vi "TEST_IR_OPO_Capture_V2.vi"(3 "AD status":bool, 5 "XPS_Address":string="192.168.254.254", 7 "laser array index":i32, 8 "OPO on?":bool, 9 "Process time":dbl format="%#_13g", 11 "Axis Speed":dbl=1.0 format="%#_13g", 12 "stop":bool, 13 "Axis Initial Parameters":T1={"Velocity (units/seconds)"=1.0, "Acceleration (units/seconds²)"=20.0, "Minimum Jerk Time (seconds)"=0.005, "Maximum Jerk Time (seconds)"=0.009} {"Maximum Jerk Time (seconds)" format="%.6e"; "Minimum Jerk Time (seconds)" format="%.6e"; "Acceleration (units/seconds²)" format="%.6e"; "Velocity (units/seconds)" format="%.6e"}, 14 "ROI Area \n(mm2)":dbl=4.035870075999999, 15 "Acceleration (units/seconds²)":dbl=20.0) -> (2 "Elapsed time":dbl)   [LabVIEW 2016]
uses:
  case selector.ctl
panel:
  in  "Commands array":string[][](array[string])=[["Group31.000000", "Group20.100000"], ["Group3-1.000000", "Group20.100000"], ["Group31.000000", "Group20.100000"], ["Group3-1.000000", "Group20.100000"], ["Group31.000000", "Group20.100000"], ["Group3-1.000000", "Group20.100000"], ["Group31.000000", "Group20.100000"], ["Group3-1.000000", "Group20.100000"], ["Group31.000000", "Group20.100000"], ["Group3-1.000000", "Group20.100000"], ["Group31.000000", "Group20.100000"], ["Group3-1.000000", "Group20.100000"]]
  in  "Laser on/off array":bool[][](array[boolean])=[[TRUE, FALSE], [TRUE, FALSE], [TRUE, FALSE], [TRUE, FALSE], [TRUE, FALSE], [TRUE, FALSE], [TRUE, FALSE], [TRUE, FALSE], [TRUE, FALSE], [TRUE, FALSE], [TRUE, FALSE], [TRUE, FALSE]]
  out "Capture Log":string="ROI Area (mm2) = 4.035870Axis 1 = 30.733482  -  Axis 2 = 11.861419\r"
  out "Axis 1 position":dbl=30.73348220365 format="%.10f"
  out "Axis 2 position":dbl=11.86141924161 format="%.10f"
  out "Initial time":timestamp=timestamp(3577899423.208551 s since 1904-01-01)
  in  "Active Positioner":string="Group2.Pos"
  out "Current Line":i32
  out "1D Laser Array":bool[](array[boolean])=[TRUE, FALSE, TRUE, FALSE, TRUE, FALSE, TRUE, FALSE, TRUE, FALSE, TRUE, FALSE, TRUE, FALSE, TRUE, FALSE, TRUE, FALSE, TRUE, FALSE, TRUE, FALSE, TRUE, FALSE]
  out "1D command array":string[](array[string])=["Group31.068", "Group20.084", "Group3-1.068", "Group20.084", "Group31.068", "Group20.084", "Group3-1.068", "Group20.084", "Group31.068", "Group20.084", "Group3-1.068", "Group20.084", "Group31.068", "Group20.084", "Group3-1.068", "Group20.084", "Group31.068", "Group20.084", "Group3-1.068", "Group20.084", "Group31.068", "Group20.084", "Group3-1.068", "Group20.084"]
  out "Current Command":string
  out "Current laser element":bool
  out "Total lines":i32
  in  "Active Axis":string="Group2"
  out "Laser on/off":bool
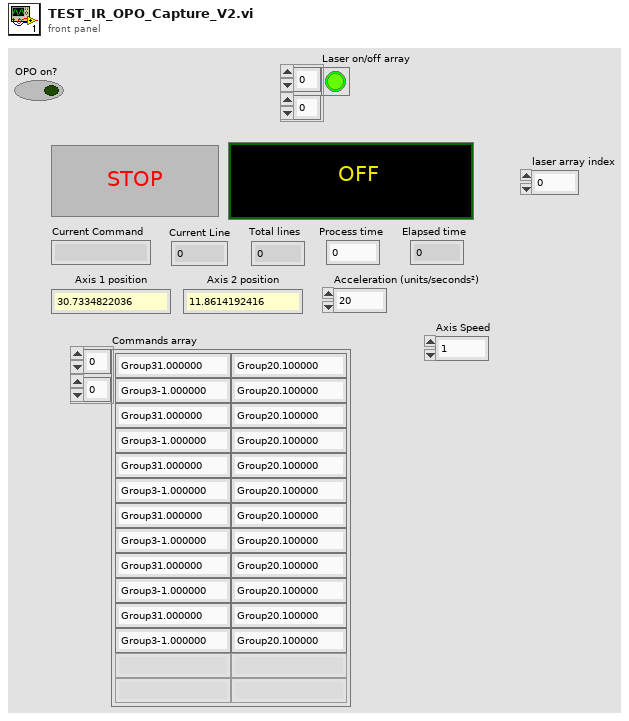
[diagram p1: front panel]
types:
  T1 = cluster{"Velocity (units/seconds)":dbl, "Acceleration (units/seconds²)":dbl, "Minimum Jerk Time (seconds)":dbl, "Maximum Jerk Time (seconds)":dbl}
  T2 = typedef "case selector.ctl" = enum16{"Initialize", "Element selection", "Laser", "Velocities", "Command", "Wait", "Exit"}
  T3 = enum16{"Initialize", "Lamp ON", "Lamp OFF", "Q-switch ON", "Q-switch OFF", "Adjust Energy", "Change Rep. Rate", "Send String"}
  T4 = enum16{"open", "replace", "create", "open or create", "replace or create", "replace or create with confirmation"}
  T5 = cluster{"connection TCP":refnum<k5>, "LogTo File":bool, "Log File refnum":refnum<file>, "no error if error log":bool}
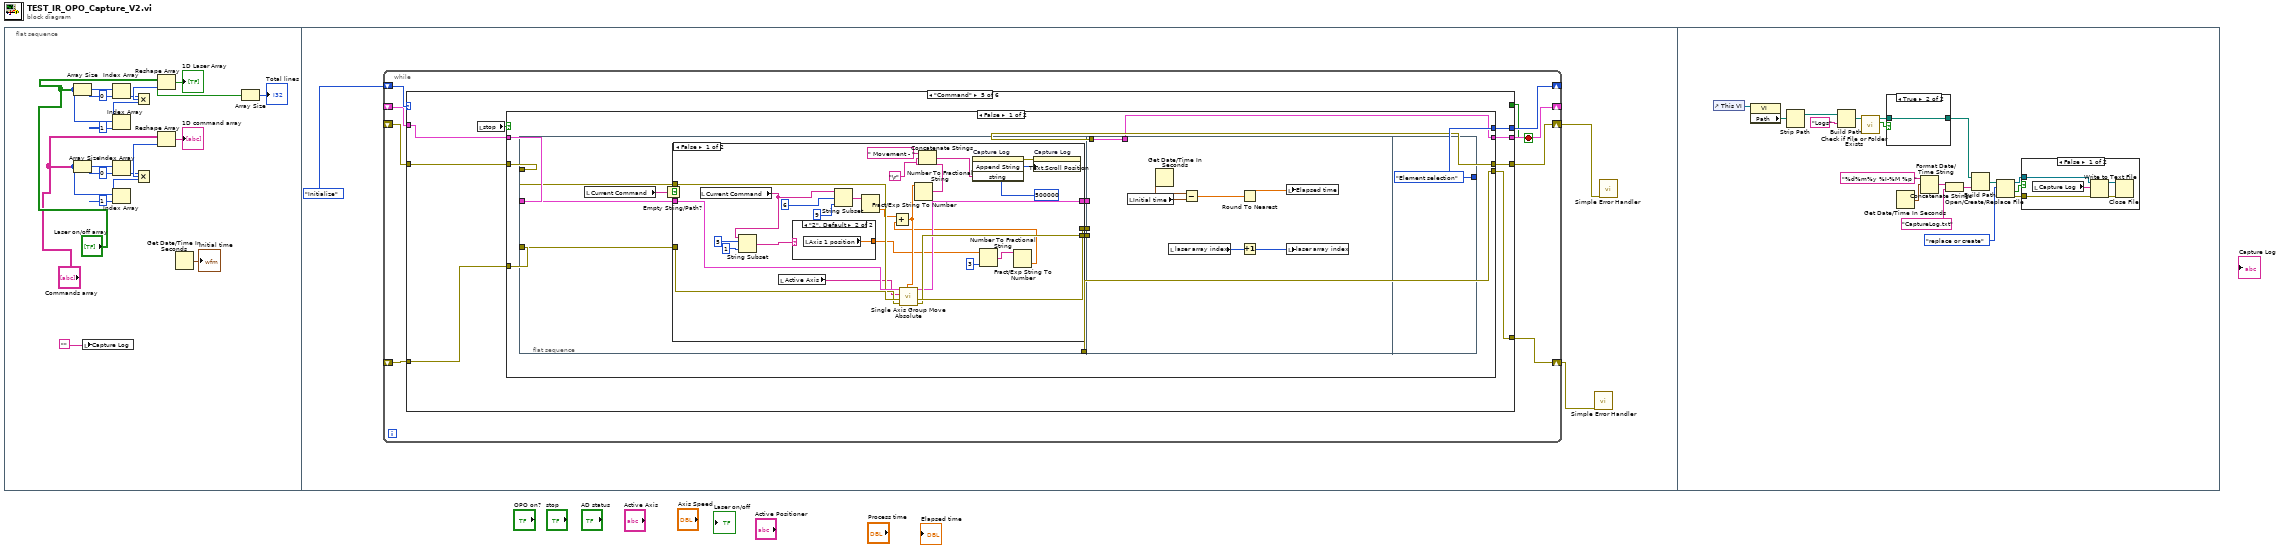
[diagram p0: block diagram]
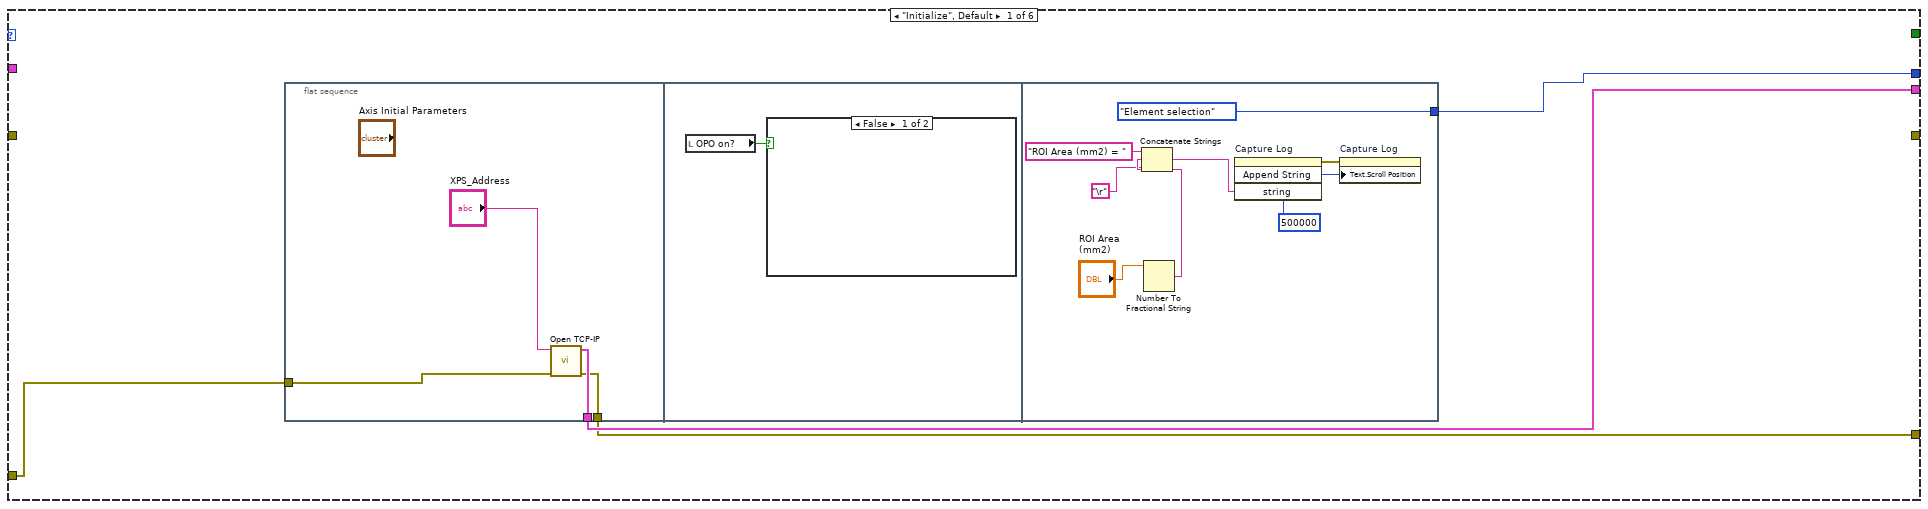
[diagram p2: hidden frame]
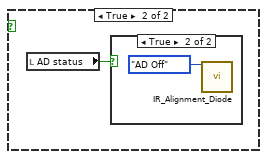
[diagram p3: hidden frame]
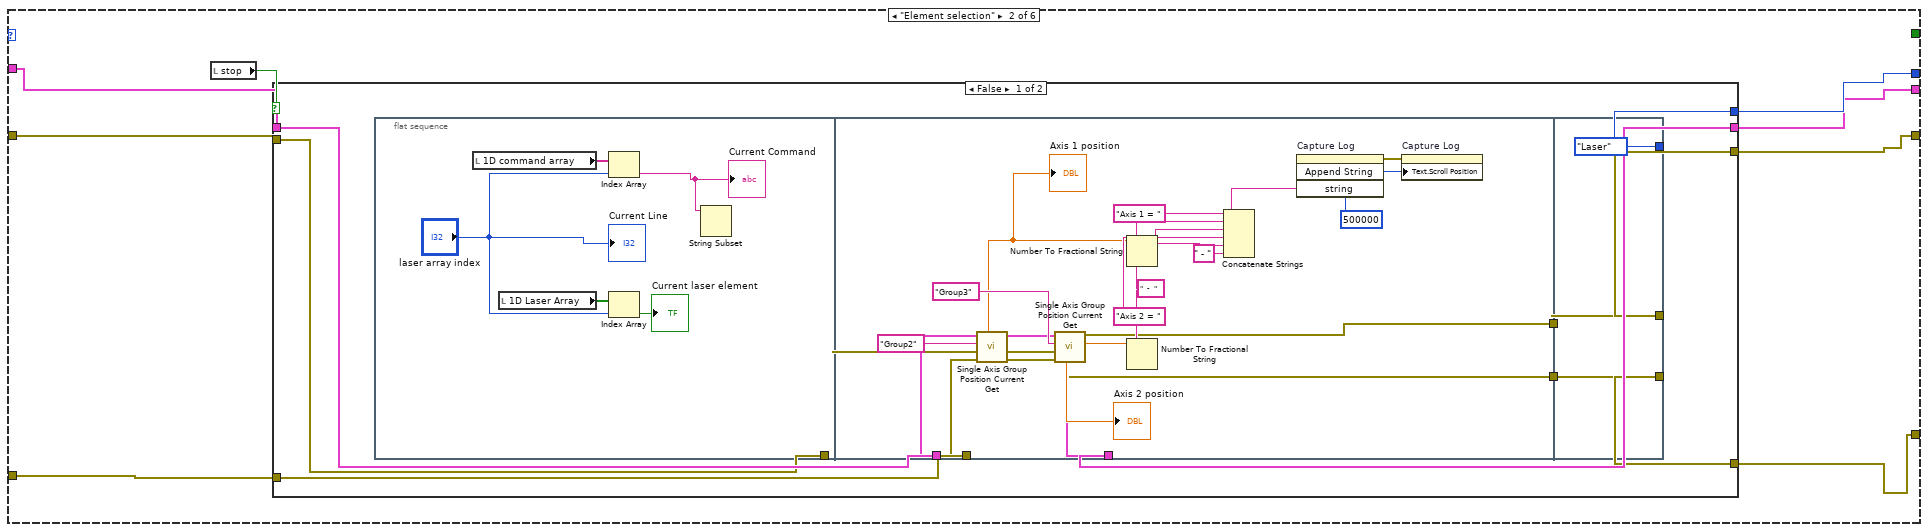
[diagram p5: hidden frame]
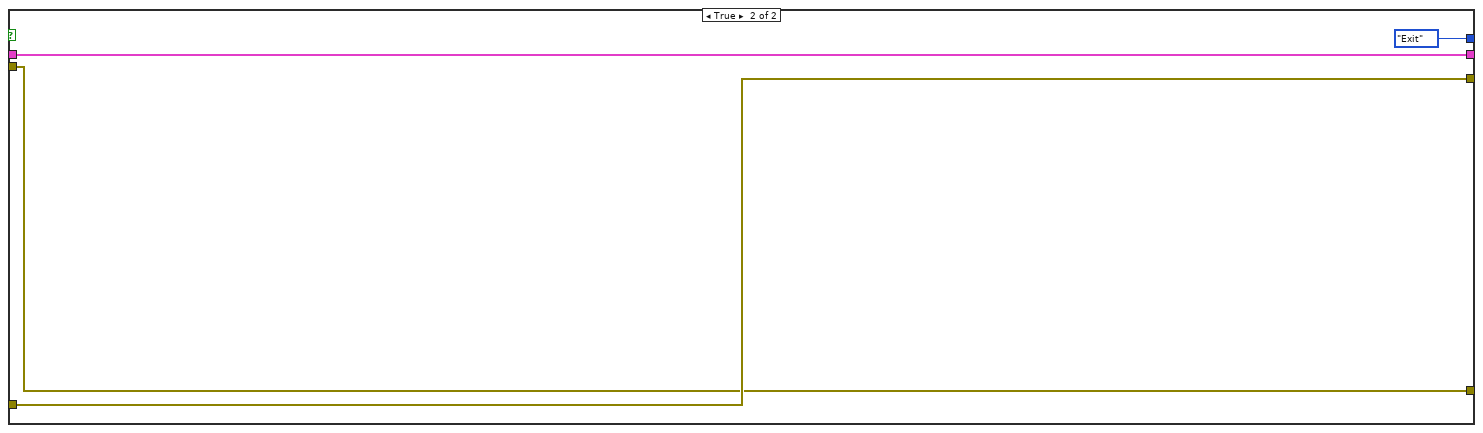
[diagram p6: hidden frame]
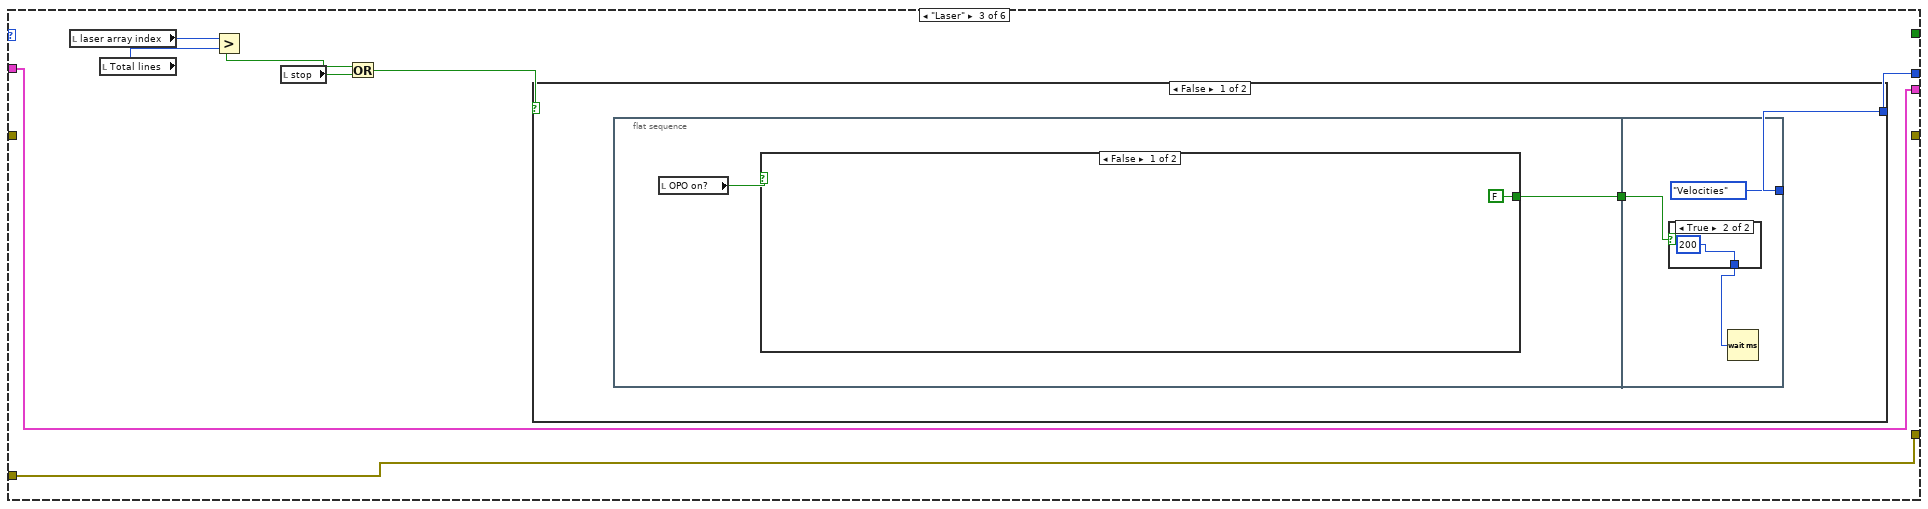
[diagram p7: hidden frame]
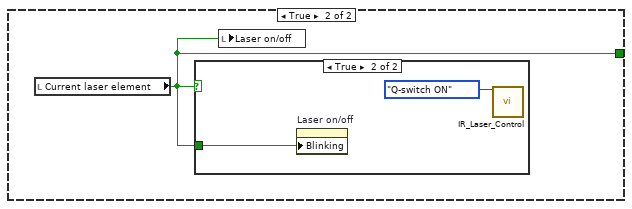
[diagram p8: hidden frame]
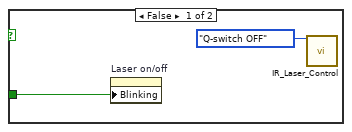
[diagram p9: hidden frame]
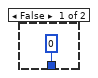
[diagram p10: hidden frame]
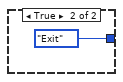
[diagram p11: hidden frame]
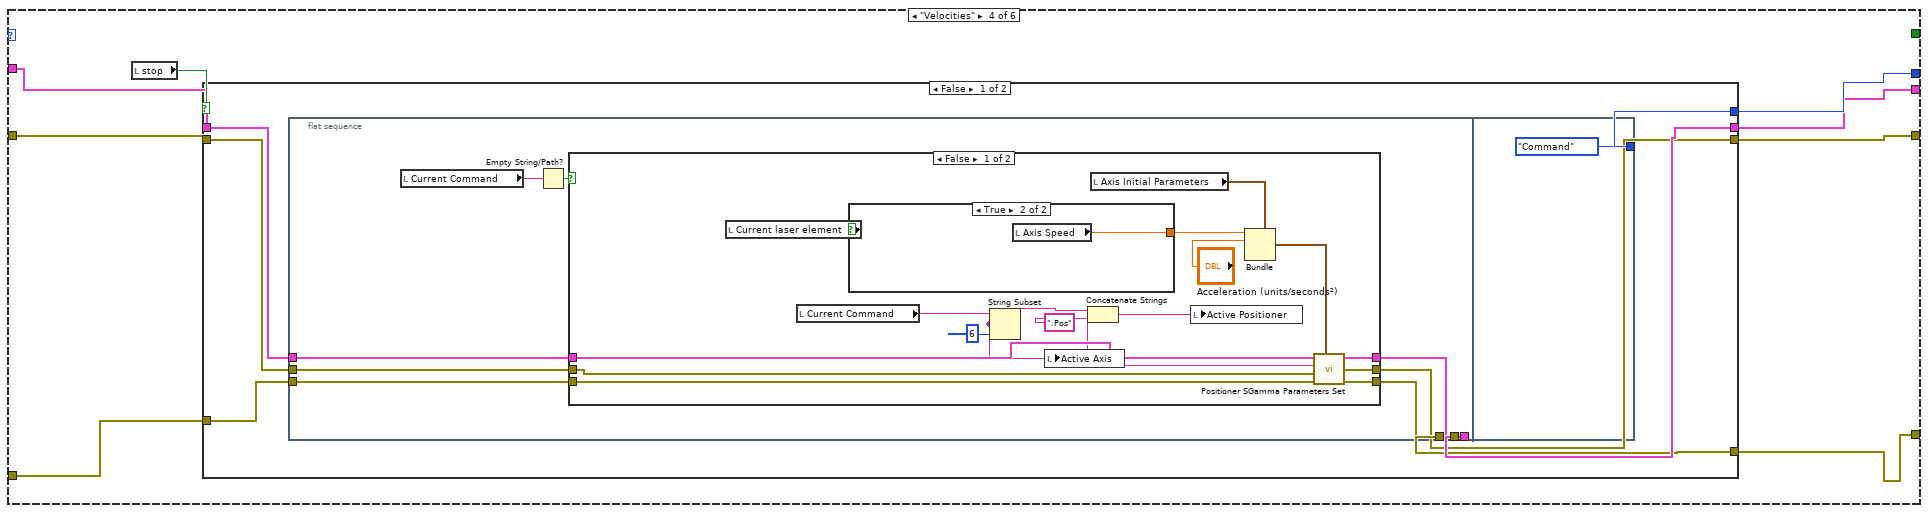
[diagram p12: hidden frame]
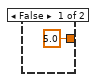
[diagram p13: hidden frame]
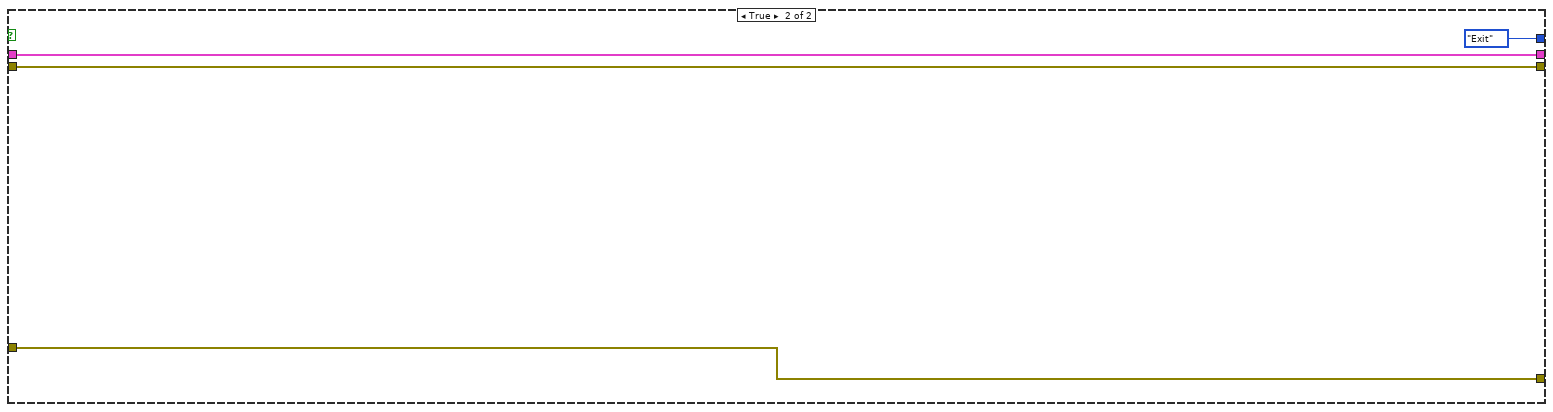
[diagram p15: hidden frame]
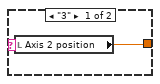
[diagram p16: hidden frame]
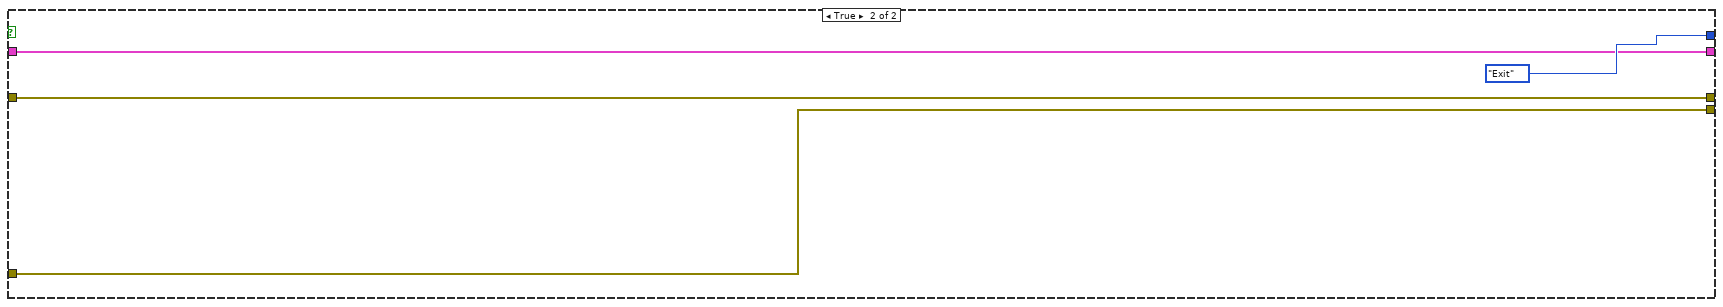
[diagram p18: hidden frame]
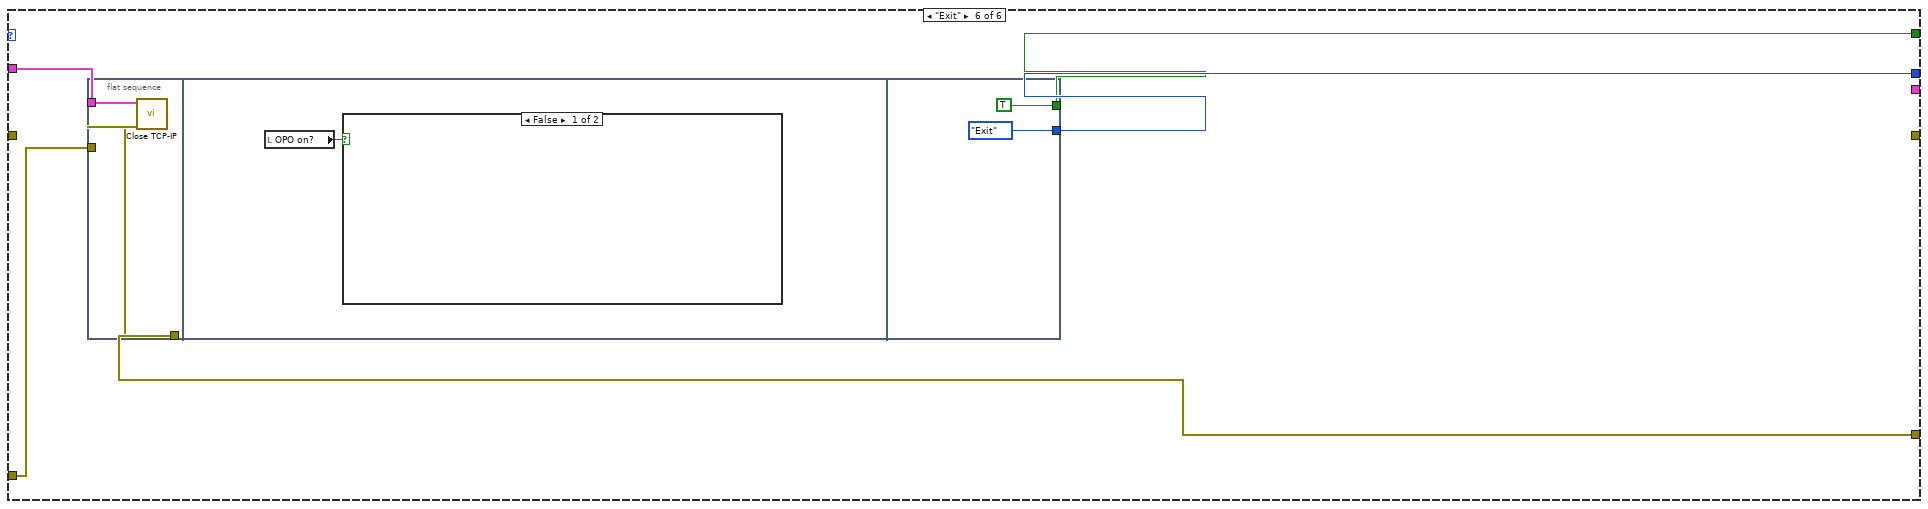
[diagram p19: hidden frame]
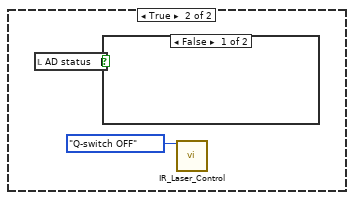
[diagram p20: hidden frame]
diagram:
  n1 = flat-sequence {
    frame #0 {
      n2 = Array Size(array="Laser on/off array") -> (size(s)=w12:i32[])
      n3 = Array Size(array="Commands array") -> (size(s)=w5:i32[])
      n4 = local write "Capture Log"("") -> ()
      n5 = Index Array(array=w12, index=0) -> (element=w15:i32)
      n6 = Index Array(array=w12, index=1) -> (element=w16:i32)
      n7 = Index Array(array=w5, index=0) -> (element=w8:i32)
      n8 = Index Array(array=w5, index=1) -> (element=w9:i32)
      n9 = Multiply(x=w15, y=w16) -> (x*y=w17:i32)
      n10 = Multiply(x=w8, y=w9) -> (x*y=w10:i32)
      n11 = Reshape Array("Laser on/off array", w17) -> (w19:bool[])
      "1D Laser Array" <- w19
      n12 = Reshape Array("Commands array", w10) -> (→"1D command array":string[])
      n13 = Get Date/Time In Seconds() -> (seconds since 1Jan1904=→"Initial time":timestamp)
      n14 = Array Size(array=w19) -> (size(s)=→"Total lines":i32)
    }
    frame #1 {
      n15 = while {
        shift-right: [w30] -> _
        shift-left: case_selector."Initialize" -> [w31]
        shift-right: [w28] -> w20
        shift-left: _ -> [w29]
        shift-right: [w27] -> _
        shift-left: _ -> [w26]
        shift-right: [w25] -> w21
        shift-left: _ -> [w24]
        stop <- w23 stop-if-true
        n16 = case shown="\"Command\"" w31 {
          tunnel: [w35 w58 w109 w133 w182 w247] -> w30
          tunnel: w29 -> [w34 w55 w108 w131 w180 w248]
          tunnel: [w32 w52 w108 w130 w179 w246] -> w28
          tunnel: [w33 w51 w102 w128 w177 _] -> w27
          tunnel: w26 -> [_ w56 w102 w129 w178 w245]
          tunnel: [_ w53 _ w127 w175 _] -> w25
          tunnel: w24 -> [_ w54 _ w126 w176 _]
          tunnel: [_ _ _ _ _ w244] -> w23
          frame "Initialize", Default {
            n17 = flat-sequence {
              tunnel: w34 -> [w38]
              tunnel: [w37] -> w33
              tunnel: [w36] -> w32
              tunnel: [case_selector."Element selection"] -> w35
              frame #0 {
                n18 = call <userlib>:"Open TCP-IP.vi"("error in (no error)"=w38, "IP address"="XPS_Address") -> ("error out"=w36:errorcluster, "Connection ID"=w37:T5)  [unwired: 7 in, 1 out]
              }
              frame #1 {
                n19 = local read "OPO on?"() -> (w40:bool)
                n20 = case shown="False" w40 {
                  frame False {
                  }
                  frame True {
                    n21 = local read "AD status"() -> (w41:bool)
                    n22 = case shown="True" w41 {
                      frame False {
                      }
                      frame True {
                        n23 = call "IR_Alignment_Diode.vi"("AD Action"=enum16{"AD Off", "AD On"}."AD Off") -> ()  [unwired: 14 in, 1 out]
                      }
                    }
                  }
                }
              }
              frame #2 {
                n24 = Number To Fractional String(number="ROI Area \n(mm2)") -> (F-format string=w46:string)  [unwired: 3 in]
                n25 = Concatenate Strings("ROI Area (mm2) = " ("string"), w46, "\r") -> (w44:string)
                n26 = invoke on="Capture Log" class="Str" method="Append String"("string"=w44) -> (error out=w48:errorcluster)  [unwired: 3 in, 3 out]
                n27 = property on="Capture Log" class="Str"(error in=w48, "Text.Scroll Position"=u32 500000) -> ()  [unwired: 1 in, 2 out]
              }
            }
          }
          frame "Element selection" {
            n28 = local read "stop"() -> (w57:bool)
            n29 = case shown="False" w57 {
              tunnel: [w64 case_selector."Exit"] -> w58
              tunnel: w56 -> [w67 w100]
              tunnel: w55 -> [w66 w99]
              tunnel: w54 -> [w65 w98]
              tunnel: [w59 w99] -> w53
              tunnel: [w61 w98] -> w52
              tunnel: [w63 w100] -> w51
              frame False {
                n30 = flat-sequence {
                  tunnel: w67 -> [w86]
                  tunnel: w66 -> [w84]
                  tunnel: w65 -> [w83]
                  tunnel: [w76] -> w63
                  tunnel: [w75] -> w62
                  tunnel: [w74] -> w60
                  tunnel: [case_selector."Laser"] -> w64
                  tunnel: w62 -> [w96]
                  tunnel: [w96] -> w61
                  tunnel: w60 -> [w95]
                  tunnel: [w95] -> w59
                  frame #0 {
                    n31 = local read "1D command array"() -> (w71:string[])
                    n32 = local read "1D Laser Array"() -> (w70:bool[])
                    n33 = Index Array(array=w71, index="laser array index") -> (element=w68:string)
                    "Current Command" <- w68
                    n34 = Index Array(array=w70, index="laser array index") -> (element=→"Current laser element":bool)
                    n35 = String Subset(string=w68) -> ()  [unwired: 2 in, 1 out]
                    "Current Line" <- "laser array index"
                  }
                  frame #1 {
                    n36 = call <userlib>:"Single Axis Group Position Current Get.vi"("error in (no error)"=w84, "XPS error in (no error)"=w83, "SingleAxis Group  Name (250 c max)"="Group2" ("Axis 1"), "connection ID in"=w86) -> ("error out"=w77:errorcluster, "XPS error out"=w78:errorcluster, "Current Position (units)"=w82:dbl, "connection ID out"=w79:T5)  [unwired: 4 in]
                    "Axis 1 position" <- w82
                    n37 = call <userlib>:"Single Axis Group Position Current Get.vi"("error in (no error)"=w77, "XPS error in (no error)"=w78, "SingleAxis Group  Name (250 c max)"="Group3" ("Axis 2"), "connection ID in"=w79) -> ("error out"=w75:errorcluster, "XPS error out"=w74:errorcluster, "Current Position (units)"=w81:dbl, "connection ID out"=w76:T5)  [unwired: 4 in]
                    "Axis 2 position" <- w81
                    n38 = Number To Fractional String(number=w82) -> (F-format string=w93:string)  [unwired: 3 in]
                    n39 = Number To Fractional String(number=w81) -> (F-format string=w91:string)  [unwired: 3 in]
                    n40 = Concatenate Strings("Axis 1 = " ("string"), w93, "  -  " ("string"), "Axis 2 = " ("string"), w91, " - " ("string")) -> (w89:string)
                    n41 = invoke on="Capture Log" class="Str" method="Append String"("string"=w89) -> (error out=w88:errorcluster)  [unwired: 3 in, 3 out]
                    n42 = property on="Capture Log" class="Str"(error in=w88, "Text.Scroll Position"=u32 500000) -> ()  [unwired: 1 in, 2 out]
                  }
                  frame #2 {
                  }
                }
              }
              frame True {
              }
            }
          }
          frame "Laser" {
            n43 = local read "laser array index"() -> (w106:i32)
            n44 = local read "Total lines"() -> (w107:i32)
            n45 = Greater?(x=w106, y=w107) -> (0:w104:bool)
            n46 = local read "stop"() -> (w105:bool)
            n47 = Or(x=w104, y=w105) -> (x .or. y?=w103:bool)
            n48 = case shown="False" w103 {
              tunnel: [w111 case_selector."Exit"] -> w109
              frame False {
                n49 = flat-sequence {
                  tunnel: [w112] -> w110
                  tunnel: [case_selector."Velocities"] -> w111
                  tunnel: w110 -> [w120]
                  frame #0 {
                    n50 = local read "OPO on?"() -> (w113:bool)
                    n51 = case shown="False" w113 {
                      tunnel: [FALSE ("Current laser element") w115] -> w112
                      frame False {
                      }
                      frame True {
                        n52 = local read "Current laser element"() -> (w115:bool)
                        n53 = case shown="True" w115 {
                          tunnel: w115 -> [w116 w118]
                          frame False {
                            n54 = property on="Laser on/off" class="Bool (strict)"("Blinking"=w116) -> ()  [unwired: 2 in, 2 out]
                            n55 = call "IR_Laser_Control.vi"("Action"=T3."Q-switch OFF") -> ()  [unwired: 14 in, 1 out]
                          }
                          frame True {
                            n56 = property on="Laser on/off" class="Bool (strict)"("Blinking"=w118) -> ()  [unwired: 2 in, 2 out]
                            n57 = call "IR_Laser_Control.vi"("Action"=T3."Q-switch ON") -> ()  [unwired: 14 in, 1 out]
                          }
                        }
                        n58 = local write "Laser on/off"(w115) -> ()
                      }
                    }
                  }
                  frame #1 {
                    n59 = case shown="True" w120 {
                      tunnel: [u32 0 ("milliseconds to wait") u32 200 ("milliseconds to wait")] -> w121
                      frame False {
                      }
                      frame True {
                      }
                    }
                    n60 = Wait (ms)(milliseconds to wait=w121) -> ()  [unwired: 1 out]
                  }
                }
              }
              frame True {
              }
            }
          }
          frame "Velocities" {
            n61 = local read "stop"() -> (w132:bool)
            n62 = case shown="False" w132 {
              tunnel: [w140 case_selector."Exit"] -> w133
              tunnel: w131 -> [w139 w173]
              tunnel: [w136 w173] -> w130
              tunnel: w129 -> [w138 w172]
              tunnel: [w137 w172] -> w128
              tunnel: [w135 w171] -> w127
              tunnel: w126 -> [w134 w171]
              frame False {
                n63 = flat-sequence {
                  tunnel: w139 -> [w146]
                  tunnel: w138 -> [w148]
                  tunnel: [w147] -> w137
                  tunnel: [w145] -> w136
                  tunnel: [w144] -> w135
                  tunnel: w134 -> [w143]
                  tunnel: [case_selector."Command"] -> w140
                  frame #0 {
                    n64 = local read "Current Command"() -> (w142:string)
                    n65 = Empty String/Path?(string/path=w142) -> (empty?=w141:bool)
                    n66 = case shown="False" w141 {
                      tunnel: w148 -> [w161 w167]
                      tunnel: [w160 w167] -> w147
                      tunnel: w146 -> [w159 w168]
                      tunnel: [w158 w168] -> w145
                      tunnel: [w153 w169] -> w144
                      tunnel: w143 -> [w152 w169]
                      frame False {
                        n67 = local read "Current laser element"() -> (w164:bool)
                        n68 = local read "Current Command"() -> (w162:string)
                        n69 = case shown="True" w164 {
                          tunnel: [5.0 w166] -> w157
                          frame False {
                          }
                          frame True {
                            n70 = local read "Axis Speed"() -> (w166:dbl)
                          }
                        }
                        n71 = String Subset(string=w162, length (rest)=6 ("length (rest)")) -> (substring=w151:string)  [unwired: 1 in]
                        n72 = local write "Active Axis"(w151) -> ()
                        n73 = Concatenate Strings(w151, ".Pos" ("string")) -> (w150:string)
                        n74 = local read "Axis Initial Parameters"() -> (w155:T1)
                        n75 = local write "Active Positioner"(w150) -> ()
                        n76 = Bundle(cluster=w155, "Velocity (units/seconds)"=w157, "Acceleration (units/seconds²)"="Acceleration (units/seconds²)") -> (w156:T1)  [unwired: 2 in]
                        n77 = call <userlib>:"Positioner SGamma Parameters Set.vi"("SGamma Parameters"=w156, "error in (no error)"=w159, "XPS error in (no error)"=w152, "Positioner Name (250 c max)"=w150, "connection ID in"=w161) -> ("error out"=w158:errorcluster, "XPS error out"=w153:errorcluster, "connection ID out"=w160:T5)  [unwired: 4 in]
                      }
                      frame True {
                      }
                    }
                  }
                  frame #1 {
                  }
                }
              }
              frame True {
              }
            }
          }
          frame "Command" {
            n78 = local read "stop"() -> (w181:bool)
            n79 = case shown="False" w181 {
              tunnel: [w186 case_selector."Exit"] -> w182
              tunnel: w180 -> [w190 w242]
              tunnel: [w184 w242] -> w179
              tunnel: w178 -> [w192 w241]
              tunnel: [w183 w241] -> w177
              tunnel: w176 -> [w189 w240]
              tunnel: [w185 w240] -> w175
              frame False {
                n80 = flat-sequence {
                  tunnel: w192 -> [w200]
                  tunnel: [w199] -> w191
                  tunnel: w190 -> [w196]
                  tunnel: w189 -> [w195]
                  tunnel: [w194] -> w188
                  tunnel: [w193] -> w187
                  tunnel: w191 -> [w230]
                  tunnel: w188 -> [w232]
                  tunnel: w187 -> [w231]
                  tunnel: [w232] -> w185
                  tunnel: [w231] -> w184
                  tunnel: [w230] -> w183
                  tunnel: [case_selector."Element selection"] -> w186
                  frame #0 {
                    n81 = local read "Current Command"() -> (w197:string)
                    n82 = Empty String/Path?(string/path=w197) -> (empty?=w198:bool)
                    n83 = case shown="False" w198 {
                      tunnel: w200 -> [w220 w229]
                      tunnel: [w221 w229] -> w199
                      tunnel: w196 -> [w218 _]
                      tunnel: w195 -> [w219 _]
                      tunnel: [w223 _] -> w194
                      tunnel: [w222 _] -> w193
                      frame False {
                        n84 = local read "Current Command"() -> (w214:string)
                        n85 = String Subset(string=w214, offset (0)=5, length (rest)=1 ("length (rest)")) -> (substring=w213:string)
                        n86 = local read "Active Axis"() -> (w217:string)
                        n87 = case shown="\"2\", Default" w213 {
                          tunnel: [w227 w228] -> w202
                          frame "3" {
                            n88 = local read "Axis 2 position"() -> (w227:dbl)
                          }
                          frame "2", Default {
                            n89 = local read "Axis 1 position"() -> (w228:dbl)
                          }
                        }
                        n90 = String Subset(string=w214, offset (0)=6, length (rest)=9 ("length (rest)")) -> (substring=w224:string)
                        n91 = Fract/Exp String To Number(string=w224) -> (number=w212:dbl)  [unwired: 3 in, 1 out]
                        n92 = Number To Fractional String(number=w202, precision (6)=i16 3) -> (F-format string=w203:string)  [unwired: 2 in]
                        n93 = Fract/Exp String To Number(string=w203) -> (number=w201:dbl)  [unwired: 3 in, 1 out]
                        n94 = Add(x=w212, y=w201) -> (x+y=w205:dbl)
                        n95 = call <userlib>:"Single Axis Group Move Absolute.vi"("Target Position (units)"=w205, "error in (no error)"=w218, "XPS error in (no error)"=w219, "SingleAxis Group  Name (250 c max)"=w217, "connection ID in"=w220) -> ("error out"=w222:errorcluster, "XPS error out"=w223:errorcluster, "connection ID out"=w221:T5)  [unwired: 4 in]
                        n96 = Number To Fractional String(number=w205) -> (F-format string=w209:string)  [unwired: 3 in]
                        n97 = Concatenate Strings(" Movement - " ("string"), w209, "\r") -> (w207:string)
                        n98 = invoke on="Capture Log" class="Str" method="Append String"("string"=w207) -> (error out=w210:errorcluster)  [unwired: 3 in, 3 out]
                        n99 = property on="Capture Log" class="Str"(error in=w210, "Text.Scroll Position"=u32 500000) -> ()  [unwired: 1 in, 2 out]
                      }
                      frame True {
                      }
                    }
                  }
                  frame #1 {
                    n100 = local read "Initial time"() -> (w235:timestamp)
                    n101 = Get Date/Time In Seconds() -> (seconds since 1Jan1904=w236:timestamp)
                    n102 = local read "laser array index"() -> (w238:i32)
                    n103 = Subtract(x=w236, y=w235) -> (x-y=w234:dbl)
                    n104 = Round To Nearest(number=w234) -> (nearest integer value=w233:dbl)
                    n105 = Increment(x=w238) -> (x+1=w237:i32)
                    n106 = local write "Elapsed time"(w233) -> ()
                    n107 = local write "laser array index"(w237) -> ()
                  }
                  frame #2 {
                  }
                }
              }
              frame True {
              }
            }
          }
          frame "Exit" {
            n108 = flat-sequence {
              tunnel: w248 -> [w250]
              tunnel: [w249] -> w246
              tunnel: w245 -> [w251]
              tunnel: [case_selector."Exit"] -> w247
              tunnel: [TRUE] -> w244
              frame #0 {
                n109 = call <userlib>:"Close TCP-IP.vi"("error in (no error)"=w250, "connection ID in"=w251) -> ("Error out"=w249:errorcluster)  [unwired: 9 in]
              }
              frame #1 {
                n110 = local read "OPO on?"() -> (w252:bool)
                n111 = case shown="False" w252 {
                  frame False {
                  }
                  frame True {
                    n112 = local read "AD status"() -> (w253:bool)
                    n113 = case shown="False" w253 {
                      frame False {
                      }
                      frame True {
                        n114 = call "IR_Alignment_Diode.vi"("AD Action"=enum16{"AD Off", "AD On"}."AD On") -> ()  [unwired: 14 in, 1 out]
                      }
                    }
                    n115 = call "IR_Laser_Control.vi"("Action"=T3."Q-switch OFF") -> ()  [unwired: 14 in, 1 out]
                  }
                }
              }
              frame #2 {
              }
            }
          }
        }
      }
      n116 = call <vilib>:"Simple Error Handler.vi"("error in (no error)"=w20) -> ()  [unwired: 4 in, 5 out]
      n117 = call <vilib>:"Simple Error Handler.vi"("error in (no error)"=w21) -> ()  [unwired: 4 in, 5 out]
    }
    frame #2 {
      n118 = control-ref of="This VI"() -> (w275:refnum<vi>)
      n119 = property class="VI"(reference=w275) -> ("Path"=w274:path)  [unwired: 1 in, 2 out]
      n120 = Strip Path(path=w274) -> (stripped path=w265:path)  [unwired: 1 out]
      n121 = Build Path(base path=w265, name or relative path="Logs") -> (appended path=w267:path)
      n122 = call <vilib>:"Check if File or Folder Exists.vi"("path"=w267) -> ("file or folder exists?"=w266:bool, "dup path"=w264:path)  [unwired: 8 in, 1 out]
      n123 = case shown="True" w266 {
        tunnel: w264 -> [w277 w278]
        tunnel: [w276 w278] -> w261
        frame False {
          n124 = Create Folder(path (use dialog)=w277) -> (created path=w276:path)  [unwired: 2 in, 2 out]
        }
        frame True {
        }
      }
      n125 = Get Date/Time In Seconds() -> (seconds since 1Jan1904=w270:timestamp)
      n126 = Format Date/Time String(time format string (%c)="%d%m%y %I-%M %p ", seconds (now)=w270) -> (date/time string=w272:string)  [unwired: 1 in]
      n127 = Concatenate Strings(w272, "CaptureLog.txt") -> (w262:string)
      n128 = Build Path(base path=w261, name or relative path=w262) -> (appended path=w263:path)
      n129 = Open/Create/Replace File(file path (use dialog)=w263, operation (0:open)=T4."replace or create") -> (refnum out=w260:refnum<file>, cancelled=w258:bool, error out=w259:errorcluster)  [unwired: 4 in]
      n130 = case shown="False" w258 {
        tunnel: w260 -> [w283 _]
        tunnel: w259 -> [w281 _]
        frame False {
          n131 = local read "Capture Log"() -> (w282:string)
          n132 = Write to Text File(file (use dialog)=w283, text=w282, error in=w281) -> (refnum out=w280:refnum<file>, error out=w279:errorcluster)  [unwired: 2 out]
          n133 = Close File(refnum=w280, error in=w279) -> ()  [unwired: 2 out]
        }
        frame True {
        }
      }
    }
  }
